vi "Begin.vi"(11 "Image Size":T1=enum."160x120") -> (0 "error out":errorcluster)   [LabVIEW 2011]
doc: "Called before other user functions, this VI is expected to open initial I/O refnums, load in file data, and do all program initialization. Notice that the <B>error out</B> terminal is simply used for data flow. Wiring it to other structures or subVIs ensures that this VI runs first."
uses:
  <vilib>/Rock Robotics/WPI/Camera/WPI_CameraImageSize.ctl
  <vilib>/Rock Robotics/SystemInterfaces/DIO/FPGA_DIOPWMChannel.ctl
  <vilib>/Rock Robotics/WPI/Joystick/WPI_JoystickDeviceEnum.ctl
  <vilib>/Rock Robotics/SystemInterfaces/DIO/FPGA_DIORelayChannel.ctl
  <vilib>/Rock Robotics/SystemInterfaces/Typedef/FPGA_TypedefDigitalModule.ctl
  <vilib>/Rock Robotics/WPI/Relay/WPI_RelayDirection.ctl
  <vilib>/Rock Robotics/SystemInterfaces/DIO/FPGA_DIOChannel.ctl
  <vilib>/Rock Robotics/WPI/RobotDrive/WPI_RobotDriveOpen2MotorWithJaguar.vi
  <vilib>/Rock Robotics/WPI/Compressor/WPI_CompressorGetSetRefNum.vi
  <vilib>/Rock Robotics/WPI/Camera/WPI_CameraWhite Balance Values.ctl
  <vilib>/Rock Robotics/WPI/Camera/WPI_CameraExposure Values.ctl
  <vilib>/Rock Robotics/WPI/Camera/WPI_CameraFrameRate.ctl
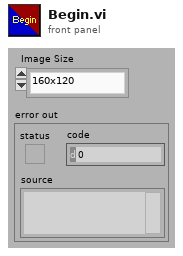
[diagram p1: front panel]
types:
  T1 = typedef "WPI_CameraImageSize.ctl" = enum16{"640x480", "320x240", "160x120"}
  T2 = typedef "FPGA_TypedefDigitalModule.ctl" = enum16{"Digital Module 1", "Digital Module 2"}
  T3 = typedef "FPGA_DIORelayChannel.ctl" = enum8{"Relay 1", "Relay 2", "Relay 3", "Relay 4", "Relay 5", "Relay 6", "Relay 7", "Relay 8", "Invalid"}
  T4 = typedef "FPGA_DIOChannel.ctl" = enum8{"DIO 1", "DIO 2", "DIO 3", "DIO 4", "DIO 5", "DIO 6", "DIO 7", "DIO 8", "DIO 9", "DIO 10", "DIO 11", "DIO 12", "DIO 13", "DIO 14", "Invalid"}
  T5 = typedef "WPI_RelayDirection.ctl" = enum16{"Both directions", "Forward only", "Reverse only"}
  T6 = typedef "WPI_JoystickDeviceEnum.ctl" = enum16{"USB 1", "USB 2", "USB 3", "USB 4", "Kinect 1", "Kinect 2"}
  T7 = typedef "FPGA_DIOPWMChannel.ctl" = enum8{"PWM 1", "PWM 2", "PWM 3", "PWM 4", "PWM 5", "PWM 6", "PWM 7", "PWM 8", "PWM 9", "PWM 10", "Invalid"}
  T8 = typedef "WPI_CameraFrameRate.ctl" = u32
  T9 = typedef "WPI_CameraExposure Values.ctl" = enum16{"Auto", "Flicker-free 50 Hz", "Flicker-free 60 Hz", "Hold current"}
  T10 = typedef "WPI_CameraWhite Balance Values.ctl" = enum16{"Auto", "Fixed indoor", "Fixed outdoor 1", "Fixed outdoor 2", "Fixed fluorescent 1", "Fixed fluorescent 2", "Hold current"}
  T11 = typedef "WPI_CameraDevRef.ctl" = cluster{"Camera Address":string, "CameraStatus":errorcluster, "Acquire Image Notifier":refnum<notifier>}
  T12 = typedef "WPI_RobotDriveDevRef.ctl" = cluster{"DevStatus":errorcluster, "Motors[]":T13[], "Square Inputs":bool, "Max Output":dbl, "Isochronous":bool}
  T13 = typedef "WPI_MotorControlDeviceRef.ctl" = cluster{"DeviceStatus":errorcluster, "Type":enum16{"PWM", "CAN"}, "PWM":cluster{"Digital Module":T2, "PWM Channel":T7, "DeadBand":T14}, "CAN":cluster{"Device Number":u8, "Control Mode":T15, "Semaphore":T16, "Max Vout":dbl}, "Invert":bool, "TransformRef":T17, "InvTransformRef":T17}
  T14 = typedef "WPI_PWMDeadband.ctl" = cluster{"Name":string, "maxPositivePwm":i32, "minPositivePwm":i32, "centerPwm":i32, "maxNegativePwm":i32, "minNegativePwm":i32, "angularRange":u16}
  T15 = typedef "WPI_CANJaguar_ControlMode.ctl" = enum8{"Percent VBus", "Current", "Speed", "Position", "Voltage"}
  T16 = typedef "Semaphore RefNum" = refnum<k1>
  T17 = typedef "WPI_PWMTransform_ConPane.ctl" = refnum<vi>
  T18 = typedef "WPI_JoystickDevRef.ctl" = cluster{"Device":T6}
  T19 = typedef "WPI_CompressorDevRef.ctl" = cluster{"DevStatus":errorcluster, "DigitalInputDevRef":T20, "RelayDevRef":T21}
  T20 = typedef "WPI_DigitalInputDevRef.ctl" = cluster{"DevStatus":errorcluster, "DIO Channel":T4, "Digital Module":T2}
  T21 = typedef "WPI_RelayDevRef.ctl" = cluster{"DevStatus":errorcluster, "Relay Channel":T3, "Digital Module":T2, "Relay Direction":T5}
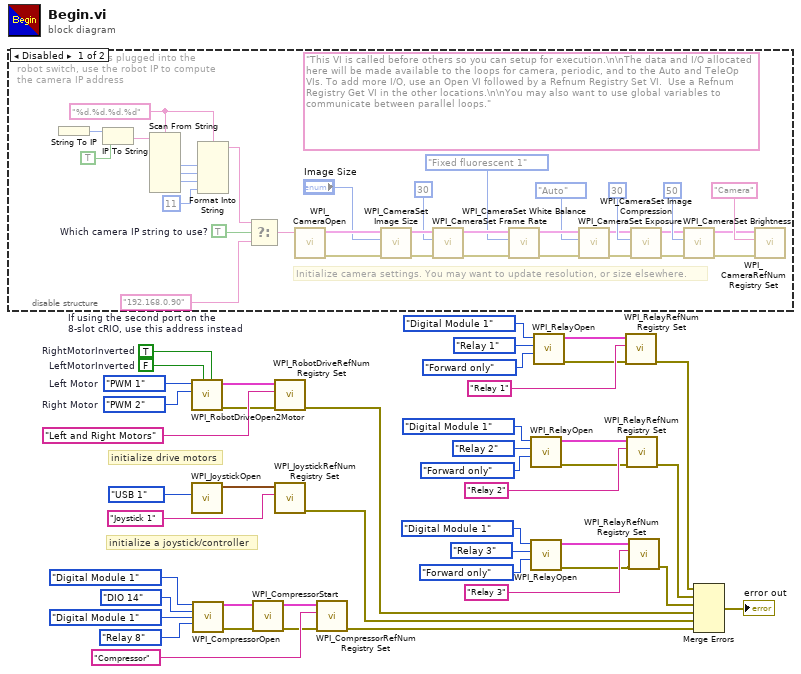
[diagram p0: block diagram]
diagram:
  w36 = FPGA_DIOPWMChannel."PWM 2"  # Right Motor
  w37 = FPGA_DIOPWMChannel."PWM 1"  # Left Motor
  w43 = FALSE  # LeftMotorInverted
  w44 = TRUE  # RightMotorInverted
  # "initialize a joystick/controller"
  # "initialize drive motors"
  n1 = disable-structure shown="Disabled" {
    frame Disabled {
      w45 = TRUE  # Which camera IP string to use?
      w49 = "%d.%d.%d.%d" ("format string")
      (unwired) "This VI is called before others so you can setup for execution.\n\nThe data and I/O allocated here will be made available to the loops for camera, periodic, and to the Auto and TeleOp VIs. To add more I/O, use an Open VI followed by a Refnum Registry Set VI.  Use a Refnum Registry Get VI in the other locations.\n\nYou may also want to use global variables to communicate between parallel loops."
      w46 = "192.168.0.90"  # If using the second port on the 8-slot cRIO, use this address instead
      # "When the camera is plugged into the\nrobot switch, use the robot IP to compute\nthe camera IP address"
      # "Initialize camera settings. You may want to update resolution, or size elsewhere."
      n2 = String To IP() -> (0:w56:u32)  [unwired: 1 in]
      n3 = IP To String(1:TRUE ("dot notation? (F)"), 2:w56) -> (0:w54:string)
      n4 = Scan From String(format string=w49, input string=w54) -> (output 1=w53:i32, output 2=w52:i32, output 3=w51:i32)  [unwired: 7 in, 3 out]
      n5 = Format Into String(format string=w49, w53, w52, w51, 11 ("Compression")) -> (resulting string=w47:string)  [unwired: 2 in, 1 out]
      n6 = Select(t=w47, s=w45, f=w46) -> (s? t:f=w48:string)
      n7 = call <vilib>:"WPI_CameraOpen.vi"("Camera Address"=w48) -> ("error out"=w68:errorcluster, "CameraDevRef"=w69:T11)  [unwired: 1 in, 8 out]
      n8 = call <vilib>:"WPI_CameraSet Image Size.vi"("error in (no error)"=w68, "Image Size"="Image Size", "CameraDevRef"=w69) -> ("error out"=w67:errorcluster, "CameraDevRef Out"=w70:T11)  [unwired: 7 out]
      n9 = call <vilib>:"WPI_CameraSet Frame Rate.vi"("error in (no error)"=w67, "Frame Rate (fps)"=T8 30, "CameraDevRef"=w70) -> ("error out"=w66:errorcluster, "CameraDevRef Out"=w72:T11)  [unwired: 7 out]
      n10 = call <vilib>:"WPI_CameraSet White Balance.vi"("error in (no error)"=w66, "White Balance"=WPI_CameraWhite_Balance_Values."Fixed fluorescent 1", "CameraDevRef"=w72) -> ("error out"=w65:errorcluster, "CameraDevRef Out"=w71:T11)  [unwired: 7 out]
      n11 = call <vilib>:"WPI_CameraSet Exposure.vi"("error in (no error)"=w65, "Exposure"=WPI_CameraExposure_Values."Auto", "CameraDevRef"=w71) -> ("error out"=w64:errorcluster, "CameraDevRef Out"=w74:T11)  [unwired: 7 out]
      n12 = call <vilib>:"WPI_CameraSet Image Compression.vi"("error in (no error)"=w64, "Compression"=30, "CameraDevRef"=w74) -> ("error out"=w63:errorcluster, "CameraDevRef Out"=w73:T11)  [unwired: 7 out]
      n13 = call <vilib>:"WPI_CameraSet Brightness.vi"("error in (no error)"=w63, "Brightness"=50, "CameraDevRef"=w73) -> ("error out"=w61:errorcluster, "CameraDevRef Out"=w62:T11)  [unwired: 7 out]
      n14 = call <vilib>:"WPI_CameraRefNum Registry Set.vi"("error in (no error)"=w61, "refnum name"="Camera", "CameraDevRef"=w62) -> ()  [unwired: 9 out]
    }
    frame Enabled {
    }
  }
  n15 = call-poly <vilib>:"WPI_RobotDriveOpen2Motor.vi"("Right Motor Inverted"=w44, "Left Motor Inverted"=w43, "Right Motor"=w36, "Left Motor"=w37) -> ("error out"=w38:errorcluster, "RobotDriveDevRef"=w42:T12)  [unwired: 1 in, 5 out]
  n16 = call <vilib>:"WPI_JoystickOpen.vi"("JoystickDevice"=WPI_JoystickDeviceEnum."USB 1") -> ("JoystickDevRef"=w40:T18)  [unwired: 10 out]
  n17 = call <vilib>:"WPI_CompressorOpen.vi"("Pressure Switch Digital Module (Module 1)"=FPGA_TypedefDigitalModule."Digital Module 1", "Pressure Switch DIO Channel"=FPGA_DIOChannel."DIO 14", "Relay Digital Module (Module 1)"=FPGA_TypedefDigitalModule."Digital Module 1", "Relay Channel"=FPGA_DIORelayChannel."Relay 8") -> ("CompressorDevRef"=w11:T19, "error out"=w10:errorcluster)  [unwired: 10 in]
  n18 = call <vilib>:"WPI_CompressorStart.vi"("error in (no error)"=w10, "CompressorDevRef"=w11) -> ("error out"=w8:errorcluster, "CompressorDevRef"=w9:T19)  [unwired: 8 in]
  n19 = call <vilib>:"WPI_RobotDriveRefNum Registry Set.vi"("error in (no error)"=w38, "refnum name"="Left and Right Motors", "RobotDriveDevRef"=w42) -> ("error out"=w3:errorcluster)  [unwired: 8 out]
  n20 = call <vilib>:"WPI_JoystickRefNum Registry Set.vi"("refnum name"="Joystick 1", "JoystickDevRef"=w40) -> ("error out"=w2:errorcluster)  [unwired: 1 in, 8 out]
  n21 = call <vilib>:"WPI_CompressorRefNum Registry Set.vi"("error in (no error)"=w8, "refnum name"="Compressor", "CompressorDevRef"=w9) -> ("error out"=w1:errorcluster)  [unwired: 7 in, 1 out]
  n22 = call <vilib>:"WPI_RelayOpen.vi"("Relay Direction"=WPI_RelayDirection."Forward only", "Relay Channel"=FPGA_DIORelayChannel."Relay 2", "Digital Module (Module 1)"=FPGA_TypedefDigitalModule."Digital Module 1") -> ("error out"=w13:errorcluster, "RelayDevRef"=w33:T21)  [unwired: 7 in]
  n23 = call <vilib>:"WPI_RelayOpen.vi"("Relay Direction"=WPI_RelayDirection."Forward only", "Relay Channel"=FPGA_DIORelayChannel."Relay 3", "Digital Module (Module 1)"=FPGA_TypedefDigitalModule."Digital Module 1") -> ("error out"=w12:errorcluster, "RelayDevRef"=w28:T21)  [unwired: 7 in]
  n24 = call <vilib>:"WPI_RelayOpen.vi"("Relay Direction"=WPI_RelayDirection."Forward only", "Relay Channel"=FPGA_DIORelayChannel."Relay 1", "Digital Module (Module 1)"=FPGA_TypedefDigitalModule."Digital Module 1") -> ("error out"=w14:errorcluster, "RelayDevRef"=w34:T21)  [unwired: 7 in]
  n25 = call <vilib>:"WPI_RelayRefNum Registry Set.vi"("error in (no error)"=w14, "refnum name"="Relay 1", "RelayDevRef"=w34) -> ("error out"=w6:errorcluster)  [unwired: 7 in, 1 out]
  n26 = call <vilib>:"WPI_RelayRefNum Registry Set.vi"("error in (no error)"=w13, "refnum name"="Relay 2", "RelayDevRef"=w33) -> ("error out"=w5:errorcluster)  [unwired: 7 in, 1 out]
  n27 = call <vilib>:"WPI_RelayRefNum Registry Set.vi"("error in (no error)"=w12, "refnum name"="Relay 3", "RelayDevRef"=w28) -> ("error out"=w4:errorcluster)  [unwired: 7 in, 1 out]
  n28 = Merge Errors(w6, w5, w4, w3, w2, w1) -> (→"error out":errorcluster)
